vi "Generator.vi"() -> ()   [LabVIEW 2021]
uses:
  LabViewZadania/Zmienna_Globalna.vi
  <vilib>/measure/NI_MAPro.lvlib
  <vilib>/measure/NI_MABase.lvlib
panel:
  in  "częstotliwość próbkowania szumu":cluster{"Fs":dbl, "#s":dbl}={"Fs"=1000.0, "#s"=1000.0} {"Fs" format="%.2p"}
  in  "seed":i32=-1
  in  "wypełnienie  (%)":dbl=50.0 format="%0.2f"
  in  "formuła sinus":string="sin(w*t)*sin(2*pi(1)*t)"
  in  "Częstotliwość próbkowania":cluster{"Fs":dbl, "#s":dbl}={"Fs"=1000.0, "#s"=1000.0} {"Fs" format="%.2p"}
  in  "Wybierz Sygnał":u16(ring) items=["SineWave", "TriangleWave", "SquareWave"]
  in  "Amplituda sygnału":dbl=16.0 format="%0.2p"
  in  "Częstotliwość":dbl=48.0
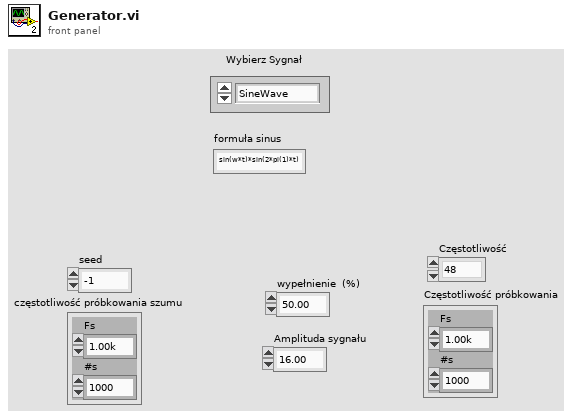
[diagram p1: front panel]
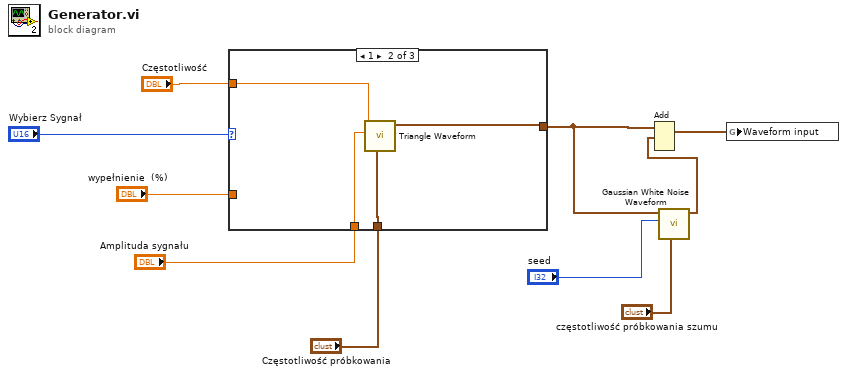
[diagram p0: block diagram]
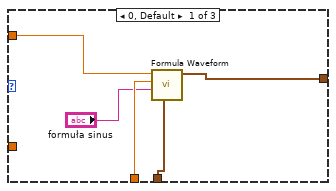
[diagram p2: hidden frame]
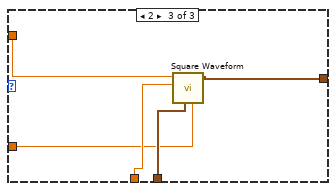
[diagram p3: hidden frame]
diagram:
  n1 = case shown="1" "Wybierz Sygnał" {
    tunnel: "Amplituda sygnału" -> [w15 w18 w23]
    tunnel: "Częstotliwość" -> [w14 w19 w24]
    tunnel: "Częstotliwość próbkowania" -> [w13 w17 w21]
    tunnel: [w11 w16 w22] -> w4
    tunnel: "wypełnienie  (%)" -> [_ _ w20]
    frame 0, Default {
      n2 = call <vilib>:"Formula Waveform.vi"("sampling info"=w13, "formula"="formuła sinus", "amplitude"=w15, "frequency"=w14) -> ("signal out"=w11:waveform(dbl))  [unwired: 6 in, 1 out]
    }
    frame 1 {
      n3 = call <vilib>:"Triangle Waveform.vi"("sampling info"=w17, "amplitude"=w18, "frequency"=w19) -> ("signal out"=w16:waveform(dbl))  [unwired: 7 in, 1 out]
    }
    frame 2 {
      n4 = call <vilib>:"Square Waveform.vi"("duty cycle (%)"=w20, "sampling info"=w21, "amplitude"=w23, "frequency"=w24) -> ("signal out"=w22:waveform(dbl))  [unwired: 6 in, 1 out]
    }
  }
  n5 = call <vilib>:"Gaussian White Noise Waveform.vi"("sampling info"="częstotliwość próbkowania szumu", "seed"="seed", "standard deviation"=w4) -> ("signal out"=w3:waveform(dbl))  [unwired: 7 in, 1 out]
  n6 = Add(1:w3, 2:w4) -> (0:w1:waveform(dbl))  [unwired: 1 in, 1 out]
  n7 = global write "Zmienna_Globalna.vi" "Waveform input"(w1) -> ()
